vi "SelectSwitchMarcoGonzalez.vi"() -> ()   [LabVIEW 2012]
panel:
  in  "?":bool
  out "Output":string
  in  "Input 2":string
  out "Strings Equal":bool
  in  "?":bool
  out "Greater than or Equal 12":bool
  in  "Input 1":dbl
  # "Marco Gonzalez\nEA 3\n02 / 23 /2017"
  # "Case 1"
  # "Case 2"
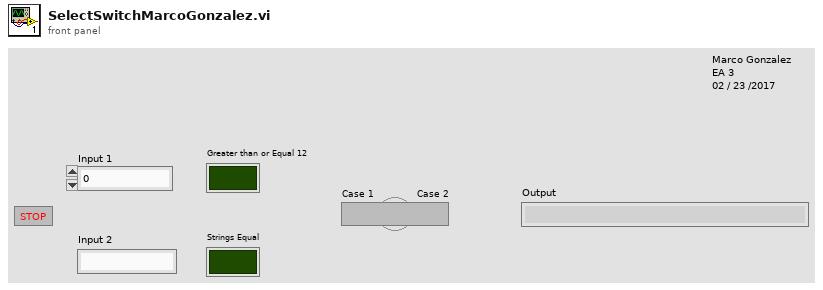
[diagram p1: front panel]
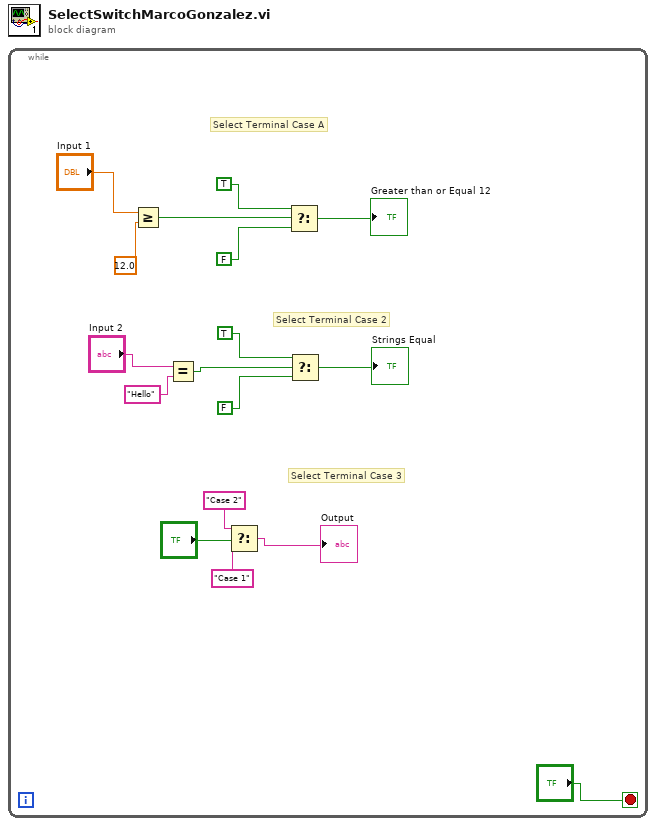
[diagram p0: block diagram]
diagram:
  n1 = while {
    stop <- "?" stop-if-true
    # "Select Terminal Case 3"
    # "Select Terminal Case 2"
    # "Select Terminal Case A"
    n2 = Greater Or Equal?(x="Input 1", y=12.0) -> (x >= y?=w15:bool)
    n3 = Equal?(x="Input 2", y="Hello") -> (x = y?=w7:bool)
    n4 = Select(t="Case 2", s="?", f="Case 1") -> (s? t:f=→"Output":string)
    n5 = Select(t=TRUE, s=w15, f=FALSE) -> (s? t:f=→"Greater than or Equal 12":bool)
    n6 = Select(t=TRUE, s=w7, f=FALSE) -> (s? t:f=→"Strings Equal":bool)
  }
